vi "Switch Pluck Data for Display.vi"(8 "error in (no error)":errorcluster, 11 "Switch Test Parameters":T1) -> (0 "error out":errorcluster, 3 "SWI Position Display":variant)   [LabVIEW 2011]
uses:
  TypeDefs/Switch Test Parameters.ctl
  TypeDefs/Switch Stimulus Parameters.ctl
  TypeDefs/Switch Type.ctl
  TypeDefs/Switch Instrument Info.ctl
  drivers/SWI/Kaelus/TypeDefs/Kaelus SWI 0206 Position Display.ctl
  drivers/SWI/Kaelus/TypeDefs/Kaelus SWI Position.ctl
  PIM/BPIM Web Engine/LIB/MODULES/SW Module/SW Tx Positions.ctl
  PIM/BPIM Web Engine/LIB/MODULES/SW Module/SW Rx Positions.ctl
  drivers/SWI/Kaelus/TypeDefs/Kaelus SWI 0309 Position Display.ctl
  drivers/SWI/Kaelus/TypeDefs/Kaelus SWI 0310 Position Display.ctl
  drivers/SWI/Sea-Level/TypeDefs/Sea-Level SWI Position Display.ctl
  drivers/SWI/Sea-Level/TypeDefs/Sea-Level SWI Position.ctl
  drivers/PFE/Kaelus/TypeDefs/Kaelus PFE Position.ctl
  drivers/PFE/Kaelus/TypeDefs/Kaelus PFE Position Display.ctl
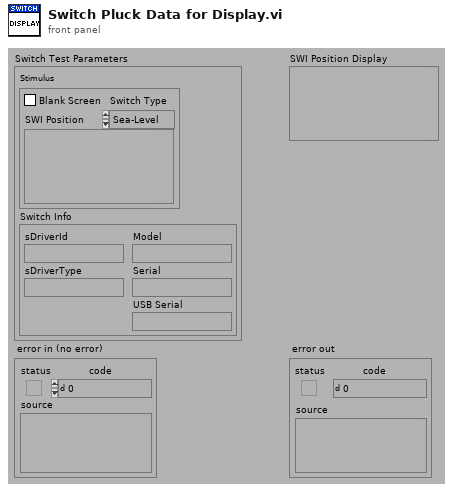
[diagram p1: front panel]
types:
  T1 = typedef "Switch Test Parameters.ctl" = cluster{"Stimulus":T2, "Switch Info":T4}
  T2 = typedef "Switch Stimulus Parameters.ctl" = cluster{"Blank Screen":bool, "SWI Position":variant, "Switch Type":T3}
  T3 = typedef "Switch Type.ctl" = enum16{"Sea-Level", "Simulator", "SI-0206-SW", "SI-0309-SW", "SI-0310-SW", "Front End"}
  T4 = typedef "Switch Instrument Info.ctl" = cluster{"sDriverId":string, "sDriverType":string, "Model":string, "Serial":string, "USB Serial":string}
  T5 = typedef "Kaelus SWI 0206 Position Display.ctl" = cluster{"Tx1":cluster{"A":bool, "B":bool, "C":bool}, "Tx2":cluster{"A":bool, "B":bool, "C":bool}}
  T6 = typedef "Kaelus SWI Position.ctl" = cluster{"Tx":T7, "Rx":T8}
  T7 = typedef "SW Tx Positions.ctl" = enum16{"TXA", "TXB", "TXC"}
  T8 = typedef "SW Rx Positions.ctl" = enum16{"RXA", "RXB", "RXC", "RXD", "RXE", "RXF"}
  T9 = typedef "Kaelus SWI 0309 Position Display.ctl" = cluster{"Tx1":cluster{"A":bool, "B":bool, "C":bool}, "Tx2":cluster{"A":bool, "B":bool, "C":bool}, "Tx2 2":cluster{"A":bool, "B":bool, "C":bool}}
  T10 = typedef "Kaelus SWI 0310 Position Display.ctl" = cluster{"Tx1":cluster{"A":bool, "B":bool}, "Tx2":cluster{"A":bool, "B":bool}, "Rx":cluster{"A":bool, "B":bool, "C":bool, "D":bool, "E":bool, "F":bool}}
  T11 = typedef "Sea-Level SWI Position Display.ctl" = cluster{"Port 1":cluster{"0":bool, "1":bool, "2":bool, "3":bool, "4":bool, "5":bool, "6":bool, "7":bool}, "Port 2":cluster{"0":bool, "1":bool, "2":bool, "3":bool, "4":bool, "5":bool, "6":bool, "7":bool}, "Port 3":cluster{"0":bool, "1":bool, "2":bool, "3":bool, "4":bool, "5":bool, "6":bool, "7":bool}, "Port 4":cluster{"0":bool, "1":bool, "2":bool, "3":bool, "4":bool, "5":bool, "6":bool, "7":bool}}
  T12 = typedef "Sea-Level SWI Position.ctl" = cluster{"Port 1 (0)":cluster{"0":bool, "1":bool, "2":bool, "3":bool, "4":bool, "5":bool, "6":bool, "7":bool}, "Port 2 (1)":cluster{"0":bool, "1":bool, "2":bool, "3":bool, "4":bool, "5":bool, "6":bool, "7":bool}, "Port 3 (2)":cluster{"0":bool, "1":bool, "2":bool, "3":bool, "4":bool, "5":bool, "6":bool, "7":bool}, "Port 4 (3)":cluster{"0":bool, "1":bool, "2":bool, "3":bool, "4":bool, "5":bool, "6":bool, "7":bool}}
  T13 = typedef "Kaelus PFE Position.ctl" = enum16{"P11 (P1 Reflected)", "P12 (P2 Through)", "P21 (P1 Through)", "P22 (P2 Reflected)"}
  T14 = typedef "Kaelus PFE Position Display.ctl" = cluster{"Tx1":cluster{"Tx":bool, "Rx":bool}, "Tx2":cluster{"Tx":bool, "Rx":bool}}
  T15 = cluster{"Boolean array[0]":bool, "Boolean array[1]":bool, "Boolean array[2]":bool}
  T16 = cluster{"Boolean array":cluster{"Boolean array[0]":bool, "Boolean array[1]":bool, "Boolean array[2]":bool}, "Boolean array":cluster{"Boolean array[0]":bool, "Boolean array[1]":bool, "Boolean array[2]":bool}}
  T17 = cluster{"Boolean array":cluster{"Boolean array[0]":bool, "Boolean array[1]":bool, "Boolean array[2]":bool}, "Boolean array":cluster{"Boolean array[0]":bool, "Boolean array[1]":bool, "Boolean array[2]":bool}, "Boolean array":cluster{"Boolean array[0]":bool, "Boolean array[1]":bool, "Boolean array[2]":bool}}
  T18 = cluster{"Boolean array[0]":bool, "Boolean array[1]":bool}
  T19 = cluster{"Boolean array[0]":bool, "Boolean array[1]":bool, "Boolean array[2]":bool, "Boolean array[3]":bool, "Boolean array[4]":bool, "Boolean array[5]":bool}
  T20 = cluster{"Boolean array":cluster{"Boolean array[0]":bool, "Boolean array[1]":bool}, "Boolean array":cluster{"Boolean array[0]":bool, "Boolean array[1]":bool}, "Boolean array":cluster{"Boolean array[0]":bool, "Boolean array[1]":bool, "Boolean array[2]":bool, "Boolean array[3]":bool, "Boolean array[4]":bool, "Boolean array[5]":bool}}
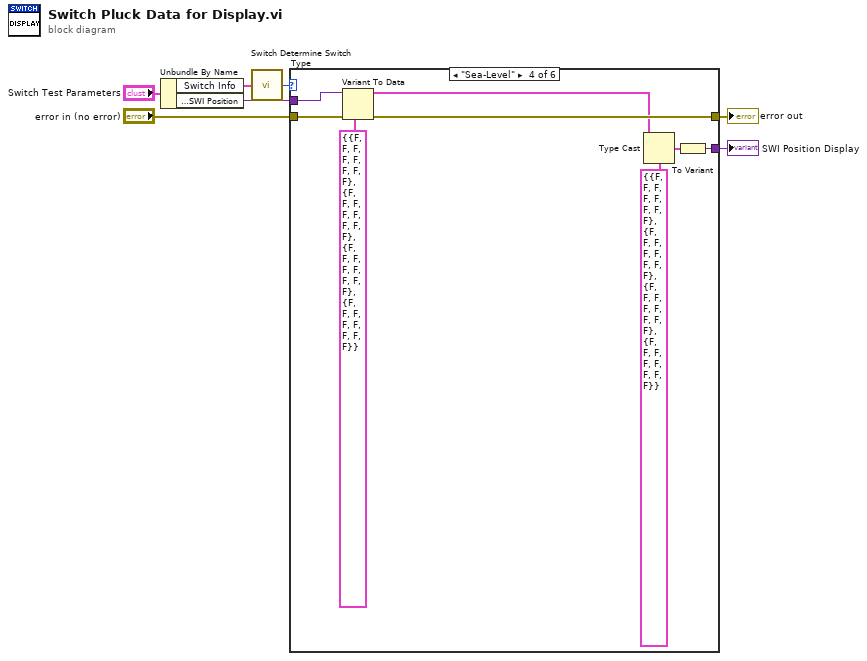
[diagram p0: block diagram]
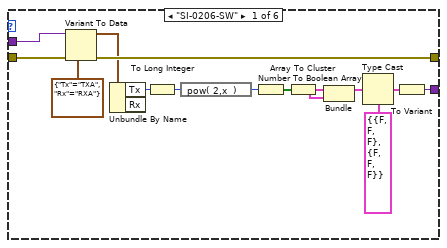
[diagram p2: hidden frame]
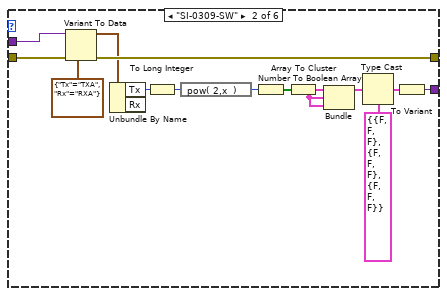
[diagram p3: hidden frame]
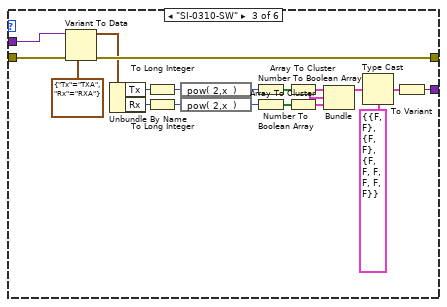
[diagram p4: hidden frame]
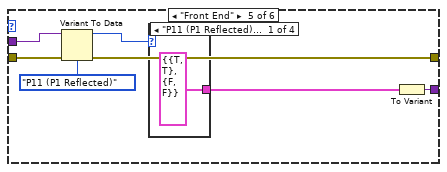
[diagram p5: hidden frame]
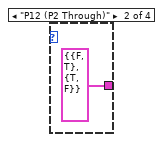
[diagram p6: hidden frame]
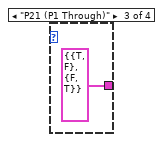
[diagram p7: hidden frame]
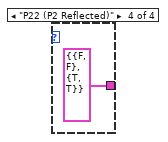
[diagram p8: hidden frame]
diagram:
  n1 = Unbundle By Name("Switch Test Parameters") -> ("Switch Info"=w3:T4, "Stimulus.SWI Position"=w1:variant)
  n2 = call "Switch Determine Switch Type.vi"("Switch Information"=w3) -> ("Switch Type"=w2:T3)  [unwired: 4 in]
  n3 = case shown="\"Sea-Level\"" w2 {
    tunnel: w1 -> [w19 w33 w52 w62 w69 _]
    tunnel: "error in (no error)" -> [w18 w32 w51 w61 w68 w74]
    tunnel: [w21 w35 w54 w60 w67 w74] -> w7
    tunnel: [w20 w34 w53 w55 w65 _] -> w6
    frame "SI-0206-SW" {
      n4 = Variant To Data(error in=w18, type=T6 {"Tx"=enum."TXA", "Rx"=enum."RXA"} ("Switch Position"), Variant=w19) -> (data=w13:T6, error out=w21:errorcluster)
      n5 = Unbundle By Name(w13) -> ("Tx"=w12:T7)  [unwired: 1 out]
      n6 = To Long Integer(number=w12) -> (32bit integer=w16:i32)
      n7 = expression code="pow( 2,x  )"(w16) -> (w15:i32)
      n8 = Number To Boolean Array(number=w15) -> (Boolean array=w14:bool[])
      n9 = Array To Cluster(array=w14) -> (cluster=w8:T15)
      n10 = Bundle("Boolean array"=w8, "Boolean array"=w8) -> (w9:T16)  [unwired: 1 in]
      n11 = Type Cast(type=T5 {"Tx1"={"A"=FALSE, "B"=FALSE, "C"=FALSE}, "Tx2"={"A"=FALSE, "B"=FALSE, "C"=FALSE}} ("Kaelus SWI Position Display"), x=w9) -> (*(type *) &x=w10:T5)
      n12 = To Variant(anything=w10) -> (Variant=w20:variant)
    }
    frame "SI-0309-SW" {
      n13 = Variant To Data(error in=w32, type=T6 {"Tx"=enum."TXA", "Rx"=enum."RXA"} ("Switch Position"), Variant=w33) -> (data=w27:T6, error out=w35:errorcluster)
      n14 = Unbundle By Name(w27) -> ("Tx"=w26:T7)  [unwired: 1 out]
      n15 = To Long Integer(number=w26) -> (32bit integer=w30:i32)
      n16 = expression code="pow( 2,x  )"(w30) -> (w29:i32)
      n17 = Number To Boolean Array(number=w29) -> (Boolean array=w28:bool[])
      n18 = Array To Cluster(array=w28) -> (cluster=w22:T15)
      n19 = Bundle("Boolean array"=w22, "Boolean array"=w22, "Boolean array"=w22) -> (w23:T17)  [unwired: 1 in]
      n20 = Type Cast(type=T9 {"Tx1"={"A"=FALSE, "B"=FALSE, "C"=FALSE}, "Tx2"={"A"=FALSE, "B"=FALSE, "C"=FALSE}, "Tx2 2"={"A"=FALSE, "B"=FALSE, "C"=FALSE}} ("Kaelus SWI Position Display"), x=w23) -> (*(type *) &x=w24:T9)
      n21 = To Variant(anything=w24) -> (Variant=w34:variant)
    }
    frame "SI-0310-SW" {
      n22 = Variant To Data(error in=w51, type=T6 {"Tx"=enum."TXA", "Rx"=enum."RXA"} ("Switch Position"), Variant=w52) -> (data=w46:T6, error out=w54:errorcluster)
      n23 = Unbundle By Name(w46) -> ("Tx"=w45:T7, "Rx"=w39:T8)
      n24 = To Long Integer(number=w45) -> (32bit integer=w49:i32)
      n25 = To Long Integer(number=w39) -> (32bit integer=w40:i32)
      n26 = expression code="pow( 2,x  )"(w49) -> (w48:i32)
      n27 = expression code="pow( 2,x  )"(w40) -> (w41:i32)
      n28 = Number To Boolean Array(number=w48) -> (Boolean array=w47:bool[])
      n29 = Number To Boolean Array(number=w41) -> (Boolean array=w42:bool[])
      n30 = Array To Cluster(array=w47) -> (cluster=w36:T18)
      n31 = Array To Cluster(array=w42) -> (cluster=w37:T19)
      n32 = Bundle("Boolean array"=w36, "Boolean array"=w36, "Boolean array"=w37) -> (w38:T20)  [unwired: 1 in]
      n33 = Type Cast(type=T10 {"Tx1"={"A"=FALSE, "B"=FALSE}, "Tx2"={"A"=FALSE, "B"=FALSE}, "Rx"={"A"=FALSE, "B"=FALSE, "C"=FALSE, "D"=FALSE, "E"=FALSE, "F"=FALSE}} ("Kaelus SWI Position Display"), x=w38) -> (*(type *) &x=w43:T10)
      n34 = To Variant(anything=w43) -> (Variant=w53:variant)
    }
    frame "Sea-Level" {
      n35 = Variant To Data(error in=w61, type=T12 {"Port 1 (0)"={"0"=FALSE, "1"=FALSE, "2"=FALSE, "3"=FALSE, "4"=FALSE, "5"=FALSE, "6"=FALSE, "7"=FALSE}, "Port 2 (1)"={"0"=FALSE, "1"=FALSE, "2"=FALSE, "3"=FALSE, "4"=FALSE, "5"=FALSE, "6"=FALSE, "7"=FALSE}, "Port 3 (2)"={"0"=FALSE, "1"=FALSE, "2"=FALSE, "3"=FALSE, "4"=FALSE, "5"=FALSE, "6"=FALSE, "7"=FALSE}, "Port 4 (3)"={"0"=FALSE, "1"=FALSE, "2"=FALSE, "3"=FALSE, "4"=FALSE, "5"=FALSE, "6"=FALSE, "7"=FALSE}} ("SWI Stimulus"), Variant=w62) -> (data=w56:T12, error out=w60:errorcluster)
      n36 = Type Cast(type=T11 {"Port 1"={"0"=FALSE, "1"=FALSE, "2"=FALSE, "3"=FALSE, "4"=FALSE, "5"=FALSE, "6"=FALSE, "7"=FALSE}, "Port 2"={"0"=FALSE, "1"=FALSE, "2"=FALSE, "3"=FALSE, "4"=FALSE, "5"=FALSE, "6"=FALSE, "7"=FALSE}, "Port 3"={"0"=FALSE, "1"=FALSE, "2"=FALSE, "3"=FALSE, "4"=FALSE, "5"=FALSE, "6"=FALSE, "7"=FALSE}, "Port 4"={"0"=FALSE, "1"=FALSE, "2"=FALSE, "3"=FALSE, "4"=FALSE, "5"=FALSE, "6"=FALSE, "7"=FALSE}} ("Sea-Level SWI Position Display"), x=w56) -> (*(type *) &x=w57:T11)
      n37 = To Variant(anything=w57) -> (Variant=w55:variant)
    }
    frame "Front End" {
      n38 = Variant To Data(error in=w68, type=Kaelus_PFE_Position."P11 (P1 Reflected)" ("SWI Stimulus"), Variant=w69) -> (data=w64:T13, error out=w67:errorcluster)
      n39 = case shown="\"P11 (P1 Reflected)\", Default" w64 {
        tunnel: [T14 {"Tx1"={"Tx"=TRUE, "Rx"=TRUE}, "Tx2"={"Tx"=FALSE, "Rx"=FALSE}} ("Switch Position") T14 {"Tx1"={"Tx"=FALSE, "Rx"=TRUE}, "Tx2"={"Tx"=TRUE, "Rx"=FALSE}} ("Switch Position") T14 {"Tx1"={"Tx"=TRUE, "Rx"=FALSE}, "Tx2"={"Tx"=FALSE, "Rx"=TRUE}} ("Switch Position") T14 {"Tx1"={"Tx"=FALSE, "Rx"=FALSE}, "Tx2"={"Tx"=TRUE, "Rx"=TRUE}} ("Switch Position")] -> w63
        frame "P11 (P1 Reflected)", Default {
        }
        frame "P12 (P2 Through)" {
        }
        frame "P21 (P1 Through)" {
        }
        frame "P22 (P2 Reflected)" {
        }
      }
      n40 = To Variant(anything=w63) -> (Variant=w65:variant)
    }
    frame "Simulator" {
    }
  }
  "error out" <- w7
  "SWI Position Display" <- w6
